vi "Arduino Focus Settings GUI.vi"(11 "Arduino Focus Settings":T1={"Port"="", "Homing Parameters"={"Direction"=TRUE, "NUMBER OF  STEPS"=13000, "SPEED STEPS/SEC"=1000, "ACC/DECEL STEPS/SEC^2"=1000, "EN/DIS?"=TRUE}, "Positions"=[], "Homed"=[]} {"Homing Parameters"."ACC/DECEL STEPS/SEC^2" max=4000; "Homing Parameters"."SPEED STEPS/SEC" min=20 max=4000 step=10}) -> (2 "Save?":bool, 3 "Settings out":T1={"Port"="", "Homing Parameters"={"Direction"=TRUE, "NUMBER OF  STEPS"=13000, "SPEED STEPS/SEC"=1000, "ACC/DECEL STEPS/SEC^2"=1000, "EN/DIS?"=TRUE}, "Positions"=[], "Homed"=[]} {"Homing Parameters"."ACC/DECEL STEPS/SEC^2" max=4000; "Homing Parameters"."SPEED STEPS/SEC" min=20 max=4000 step=10})   [LabVIEW 2022 SP3, in "ArduinoFocus.lvclass"]
uses:
  ArduinoFocus.lvclass
  ArduinoFocus.lvclass/ArduinoFocus.ctl
  Motor Control Driver/arduino Motor Control cluster Command.ctl
  Arduino Focus cluster Settings.ctl
panel:
  in  "Cancel Button":bool
  in  "OK Button":bool
  in  "Port":refnum<visa-resource-name>
  in  "Homing Parameters":T2={"Direction"=TRUE, "NUMBER OF  STEPS"=13000, "SPEED STEPS/SEC"=1000, "ACC/DECEL STEPS/SEC^2"=1000, "EN/DIS?"=TRUE} {"ACC/DECEL STEPS/SEC^2" max=4000; "SPEED STEPS/SEC" min=20 max=4000 step=10}
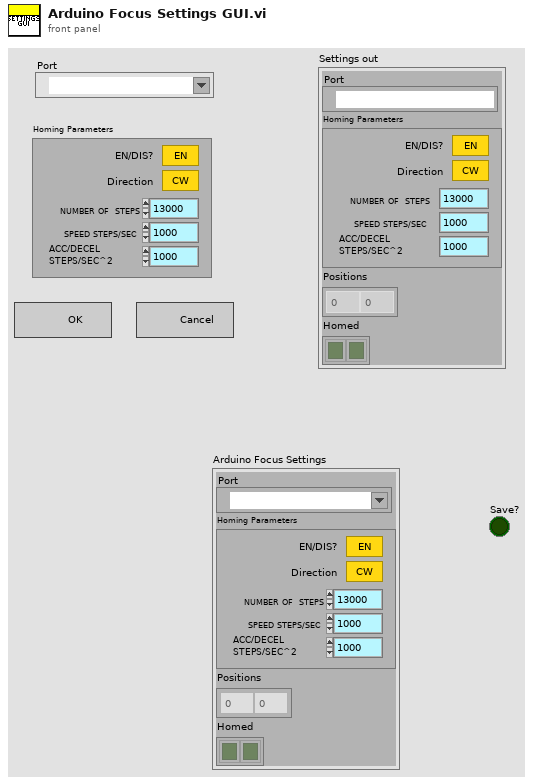
[diagram p1: front panel]
types:
  T1 = typedef "ArduinoFocus.lvclass/Arduino Focus cluster Settings.ctl" = cluster{"Port":refnum<visa-resource-name>, "Homing Parameters":T2, "Positions":i32[], "Homed":bool[]}
  T2 = typedef "arduino Motor Control cluster Command.ctl" = cluster{"Direction":bool, "NUMBER OF  STEPS":u32, "SPEED STEPS/SEC":u16, "ACC/DECEL STEPS/SEC^2":u16, "EN/DIS?":bool}
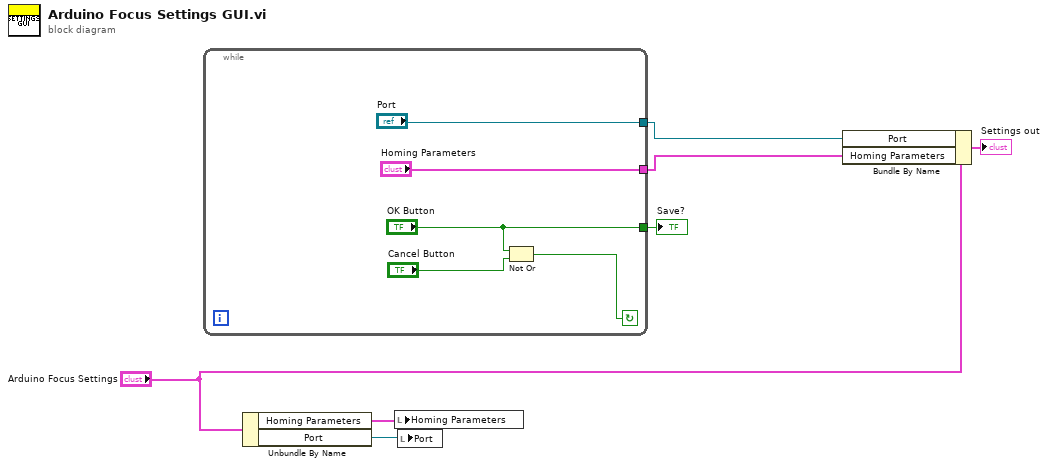
[diagram p0: block diagram]
diagram:
  n1 = while {
    tunnel: ["Homing Parameters"] -> w2
    tunnel: ["Port"] -> w3
    tunnel: ["OK Button"] -> w5
    stop <- w11 continue-if-true
    n2 = Not Or(1:"Cancel Button", 2:"OK Button") -> (0:w11:bool)
  }
  "Save?" <- w5
  n3 = Unbundle By Name("Arduino Focus Settings") -> ("Homing Parameters"=w6:T2, "Port"=w7:refnum<visa-resource-name>)
  n4 = local write "Homing Parameters"(w6) -> ()
  n5 = local write "Port"(w7) -> ()
  n6 = Bundle By Name(cluster="Arduino Focus Settings", "Port"=w3, "Homing Parameters"=w2) -> (→"Settings out":T1)
